vi "Enclose in Structure - Core.vi"(8 "error in":errorcluster, 9 "Structure Type":T1, 10 "T: Replace / F: Enclose":bool, 11 "VI in":refnum<vi>) -> (0 "error out":errorcluster, 3 "VI out":refnum<vi>)   [LabVIEW 2020]
uses:
  Enclose in Structure - Structure Type.ctl
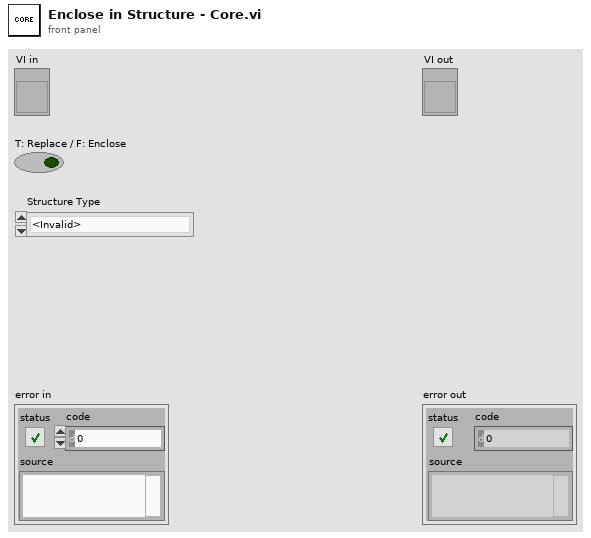
[diagram p1: front panel]
types:
  T1 = typedef "Enclose in Structure - Structure Type.ctl" = enum16{"<Invalid>", "For Loop", "While Loop", "Timed Loop", "Timed Sequence", "Case Structure", "Event Structure", "In Place Element Structure", "Flat Sequence", "Diagram Disable Structure", "Conditional Disable Structure", "Type Specialization Structure"}
  T2 = typedef "LVRectTypeDef.ctl" = cluster{"Left":i16, "Top":i16, "Right":i16, "Bottom":i16}
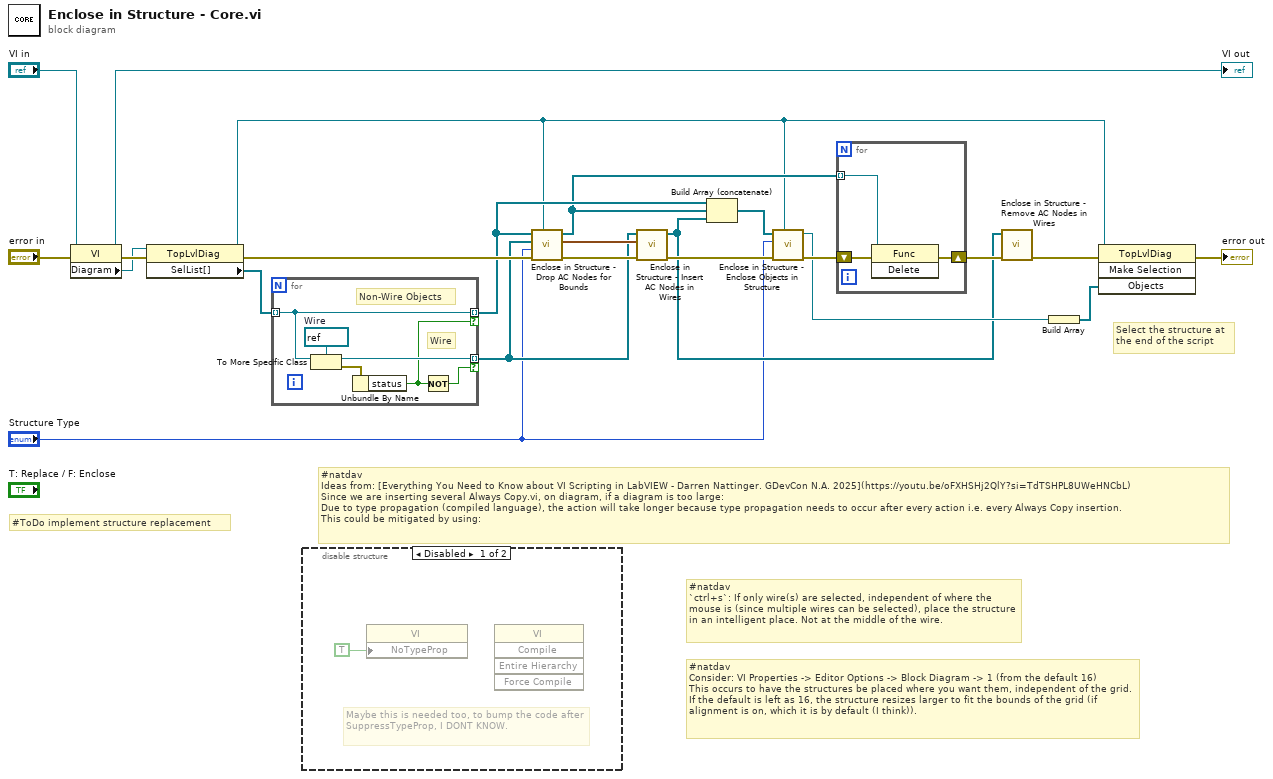
[diagram p0: block diagram]
diagram:
  # "#natdav\n`ctrl+s`: If only wire(s) are selected, independent of where the mouse is (since multiple wires can be selected), place the structure in an intelligent place. Not at the middle of the wire."
  # "#natdav\nConsider: VI Properties -> Editor Options -> Block Diagram -> 1 (from the default 16)\nThis occurs to have the structures be placed where you want them, independent of the grid. If the default is left as 16, the structure resizes larger to fit the bounds of the grid (if alignment is on, which it is by default (I think))."
  # "#natdav\nIdeas from: [Everything You Need to Know about VI Scripting in LabVIEW - Darren Nattinger. GDevCon N.A. 2025](https://youtu.be/oFXHSHj2QlY?si=TdTSHPL8UWeHNCbL)\nSince we are inserting several Always Copy.vi, on diagram, if a diagram is too large:\nDue to type propagation (compiled language), the action will take longer because type propagation needs to occur after every action i.e. every Always Copy insertion.\nThis could be mitigated by using:"
  # "Select the structure at the end of the script"
  # "#ToDo implement structure replacement"
  n1 = property class="VI"(reference="VI in", error in="error in") -> (reference out=→"VI out":refnum<vi>, error out=w18:errorcluster, "Diagram"=w17:refnum<vi>)
  n2 = property class="TopLvlDiag"(reference=w17, error in=w18) -> (reference out=w5:refnum<vi>, error out=w21:errorcluster, "SelList[]"=w19:refnum<vi>[])
  n3 = for {
    tunnel: w19 -> [w26] mode=indexing
    tunnel: [w27] -> w11 mode=indexing if=w24
    tunnel: [w26] -> w10 mode=indexing if=w25
    w29 = refnum<vi> refnum  # Wire
    # "Wire"
    # "Non-Wire Objects"
    n4 = To More Specific Class(target class=w29, reference=w26) -> (specific class reference=w27:refnum<vi>, error out=w28:errorcluster)  [unwired: 1 in]
    n5 = Unbundle By Name(w28) -> ("status"=w25:bool)
    n6 = Not(x=w25) -> (.not. x?=w24:bool)
  }
  n7 = disable-structure shown="Disabled" {
    frame Disabled {
      # "Maybe this is needed too, to bump the code after SuppressTypeProp, I DONT KNOW."
      n8 = property class="VI"("NoTypeProp"=TRUE ("Suppress Type Prop")) -> ()  [unwired: 2 in, 2 out]
      n9 = invoke class="VI" method="Compile"() -> ()  [unwired: 5 in, 5 out]
    }
    frame Enabled {
    }
  }
  n10 = call "Enclose in Structure - Drop AC Nodes for Bounds.vi"("Top Level Diagram"=w5, "error in"=w21, "Structure Type"="Structure Type", "Wires"=w11, "Non-Wire Objects"=w10) -> ("error out"=w15:errorcluster, "Bounds"=w12:T2, "Always Copy Nodes"=w8:refnum<vi>[])  [unwired: 4 in]
  n11 = call "Enclose in Structure - Insert AC Nodes in Wires.vi"("error in"=w15, "Bounds"=w12, "Wires"=w11) -> ("error out"=w22:errorcluster, "Always Copy Nodes"=w2:refnum<vi>[])  [unwired: 7 in]
  n12 = Build Array (concatenate)(w10, w8, w2) -> (w13:refnum<vi>[])
  n13 = call "Enclose in Structure - Enclose Objects in Structure.vi"("Top Level Diagram"=w5, "error in"=w22, "Structure Type"="Structure Type", "Objects"=w13) -> ("error out"=w14:errorcluster, "Structure"=w3:refnum<vi>)  [unwired: 6 in]
  n14 = for {
    shift-right: [w32] -> w23
    shift-left: w14 -> [w33]
    tunnel: w8 -> [w31] mode=indexing
    n15 = invoke class="Func" method="Delete"(reference=w31, error in=w33) -> (error out=w32:errorcluster)  [unwired: 1 in, 2 out]
  }
  n16 = call "Enclose in Structure - Remove AC Nodes in Wires.vi"("error in"=w23, "Always Copy Nodes"=w2) -> ("error out"=w7:errorcluster)  [unwired: 9 in]
  n17 = Build Array(w3) -> (w4:refnum<vi>[])
  n18 = invoke class="TopLvlDiag" method="Make Selection"(reference=w5, error in=w7, "Objects"=w4) -> (error out=→"error out":errorcluster)  [unwired: 1 in, 3 out]
